vi "ADCP_read_packet_from_serial_port_emulator.vi"(0 "ADCP In":refnum<class "ADCP.lvclass">, 11 "error in (no error)":errorcluster) -> (1 "Checksum Valid ?":bool, 2 "Packet Type":T1(ring), 3 "Packet_Priority":enum16{"LOW", "HIGH"}(ring), 4 "ADCP out":refnum<class "ADCP.lvclass">, 6 "Received Packet":u8[](array[numeric]), 8 "Packet node ID":u8, 10 "Packet frame ID":u8, 15 "error out":errorcluster)   [LabVIEW 2017, in "ADCP.lvclass"]
uses:
  ADCP.lvclass
  ADCP.lvclass/ADCP.ctl
  <vilib>/Instr/_visa.llb/VISA Flush IO Buffer Mask.ctl
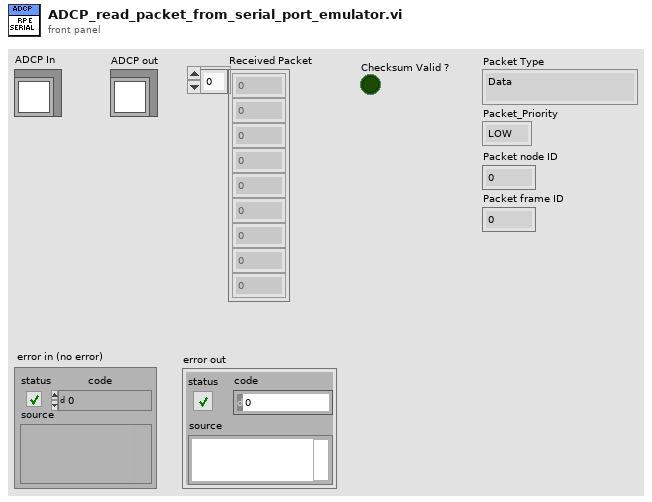
[diagram p1: front panel]
types:
  T1 = enum16{"Data", "Connection Management", "Remote Request", "Error and status", "INVALID"}
  T2 = typedef "VISA Flush IO Buffer Mask.ctl" = u16
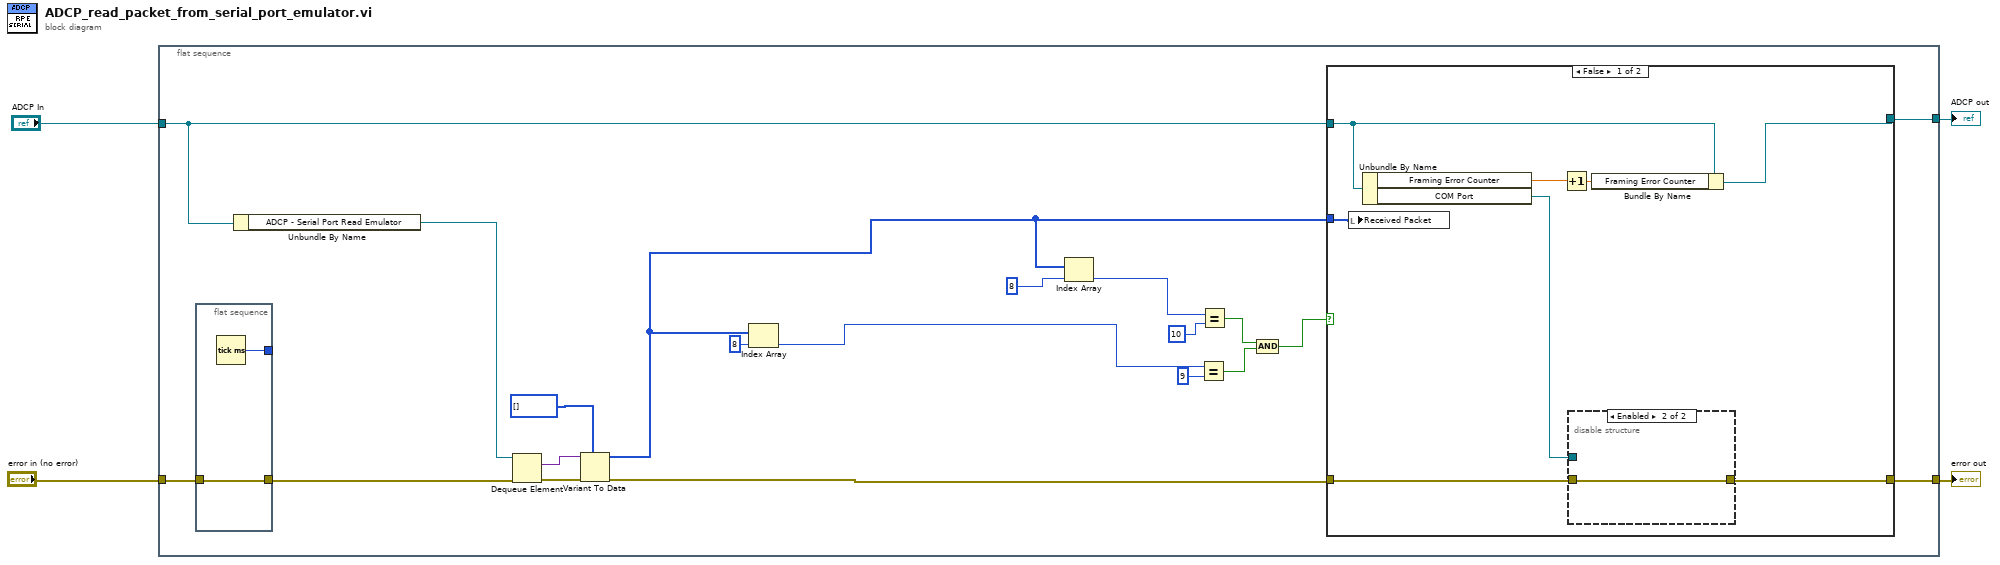
[diagram p0: block diagram]
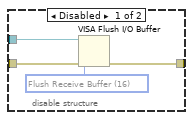
[diagram p2: hidden frame]
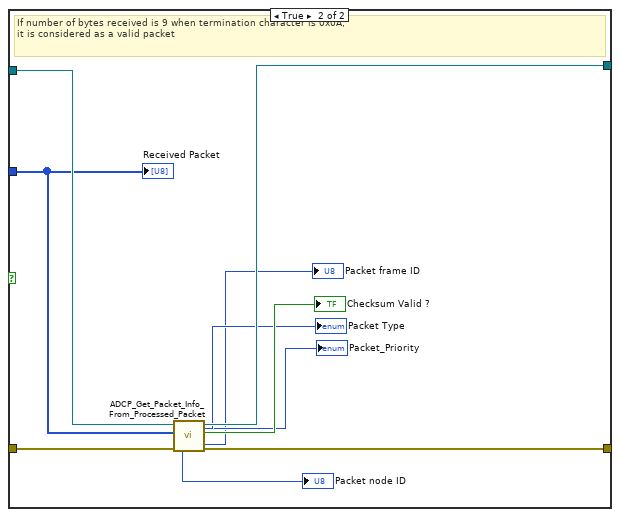
[diagram p3: hidden frame]
diagram:
  n1 = flat-sequence {
    tunnel: "ADCP In" -> [w21]
    tunnel: "error in (no error)" -> [w24]
    tunnel: [w22] -> w2
    tunnel: [w20] -> w1
    frame #0 {
      n2 = flat-sequence {
        tunnel: w24 -> [w49]
        tunnel: [w49] -> w13
        tunnel: [w48] -> _
        frame #0 {
          n3 = Tick Count (ms)() -> (millisecond timer value=w48:u32)
        }
      }
      n4 = Unbundle By Name(w21) -> ("ADCP - Serial Port Read Emulator"=w12:refnum<queue>)
      n5 = Dequeue Element(queue=w12, error in (no error)=w13) -> (element=w11:variant, error out=w10:errorcluster)  [unwired: 1 in, 2 out]
      n6 = Variant To Data(error in=w10, type=u8[] [], Variant=w11) -> (data=w7:u8[], error out=w8:errorcluster)
      n7 = Index Array(array=w7, index=8) -> (element=w5:u8)
      n8 = Index Array(array=w7, index=8) -> (element=w18:u8)
      n9 = Equal?(x=w5, y=9) -> (x = y?=w16:bool)
      n10 = Equal?(x=w18, y=10) -> (x = y?=w17:bool)
      n11 = And(x=w17, y=w16) -> (x .and. y?=w14:bool)
      n12 = case shown="False" w14 {
        tunnel: w8 -> [w27 w47]
        tunnel: w7 -> [w28 w44]
        tunnel: [w26 w46] -> w22
        tunnel: w21 -> [w30 w45]
        tunnel: [w29 w43] -> w20
        frame False {
          n13 = local write "Received Packet"(w28) -> ()
          n14 = Unbundle By Name(w30) -> ("Framing Error Counter"=w32:dbl, "COM Port"=w25:refnum<visa-resource-name>)
          n15 = Increment(x=w32) -> (x+1=w31:dbl)
          n16 = disable-structure shown="Enabled" {
            disable-tunnel: w27 -> [w36 w37]
            disable-tunnel: [w35 w37] -> w26
            disable-tunnel: w25 -> [w34 _]
            frame Disabled {
              w33 = T2 16 items=["Flush Receive Buffer"=16, "Write Transmit Buffer to Device"=32, "Flush Receive Buffer (No I/O)"=64, "Flush Transmit Buffer"=128] ("Mask")
              n17 = VISA Flush I/O Buffer(VISA resource name=w34, mask (16)=w33, error in (no error)=w36) -> (error out=w35:errorcluster)  [unwired: 1 out]
            }
            frame Enabled {
            }
          }
          n18 = Bundle By Name(cluster=w30, "Framing Error Counter"=w31) -> (w29:refnum<class "ADCP.lvclass">)
        }
        frame True {
          # "If number of bytes received is 9 when termination character is 0x0A,\nit is considered as a valid packet"
          n19 = call "ADCP_Get_Packet_Info_From_Processed_Packet.vi"("error in (no error)"=w47, "Processed Packet"=w44, "ADCP in"=w45) -> ("error out"=w46:errorcluster, "Checksum Valid ?"=→"Checksum Valid ?":bool, "ADCP out"=w43:refnum<class "ADCP.lvclass">, "Packet frame ID"=→"Packet frame ID":u8, "Packet Type"=→"Packet Type":T1, "Packet node ID"=→"Packet node ID":u8, "Packet_Priority"=→"Packet_Priority":enum16{"LOW", "HIGH"})  [unwired: 2 in]
          "Received Packet" <- w44
        }
      }
    }
  }
  "error out" <- w2
  "ADCP out" <- w1
